vi "γ能量测量实验.vi"() -> ()   [LabVIEW 2014]
panel:
  in  "放大倍数":dbl min=0.0 max=2.0
  in  "按钮_提示":bool caption="提示"
  in  "选项卡控件 实验步骤":T1(tab)
  in  "选项卡控件":enum32{"选项卡 3", "选项卡 1", "选项卡 2", "选项卡 4"}(tab)
  in  "放射源":string(combo)
  in  "按钮_退出":bool
  in  "按钮_开始测量":bool
  in  "按钮_加载高压":bool
  in  "按钮_放置放射源":bool
  in  "按钮_打开多道":bool
  out "高压输入":bool
  out "0-1KV":dbl(knob) scale=0.0..1.0
  out "信号输出指示":bool caption="信号输出"
  in  "按钮_恢复仪器状态":bool
  out "退出":bool
  out "信号输出":bool
  out "是否放置放射源":bool
  in  "脉冲间隔时间":i16
  in  "数组_各放射源初始计数率":dbl[](array[numeric])
  # "实验：γ能谱测量实验"
  # "实验仪器"
  # "实验原理"
  # "实验步骤"
  # "操作面板"
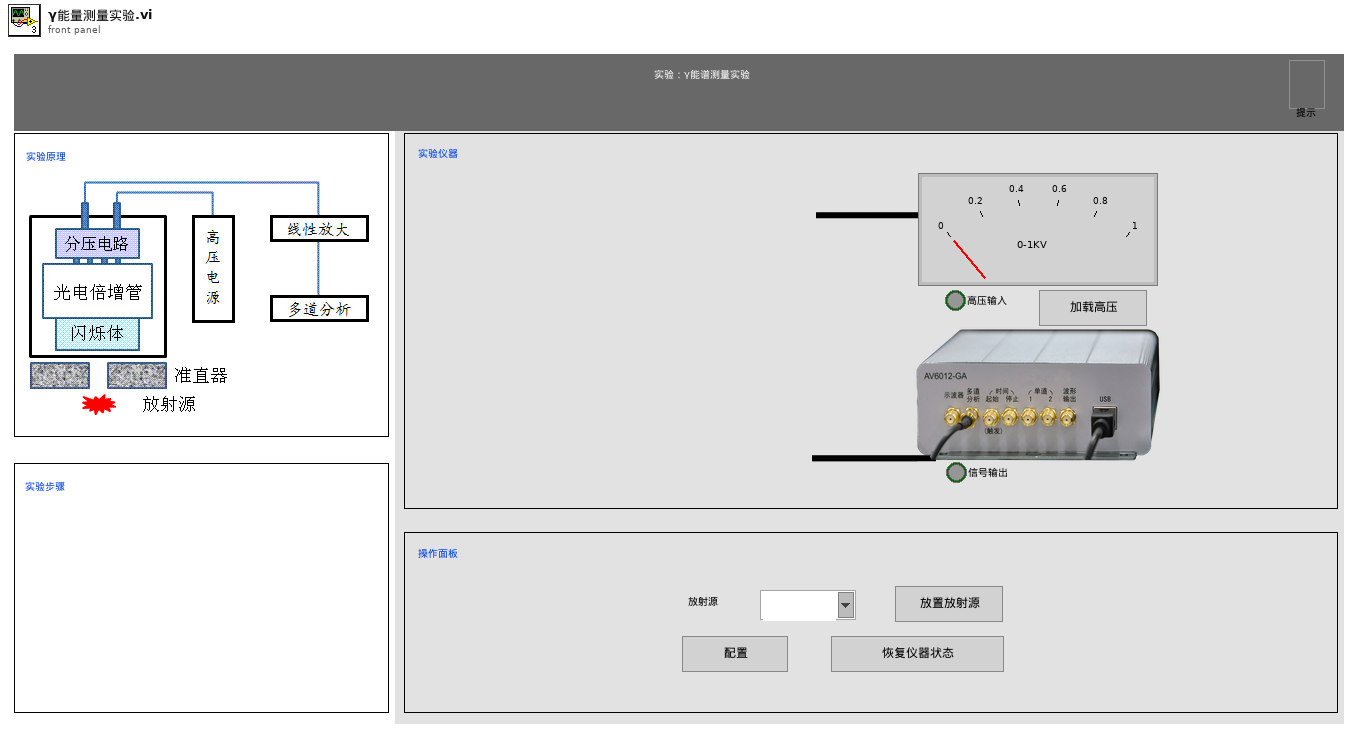
[diagram p1: front panel]
types:
  T1 = enum32{"选项卡 1", "选项卡 2", "选项卡 3", "选项卡 4", "选项卡 5"}
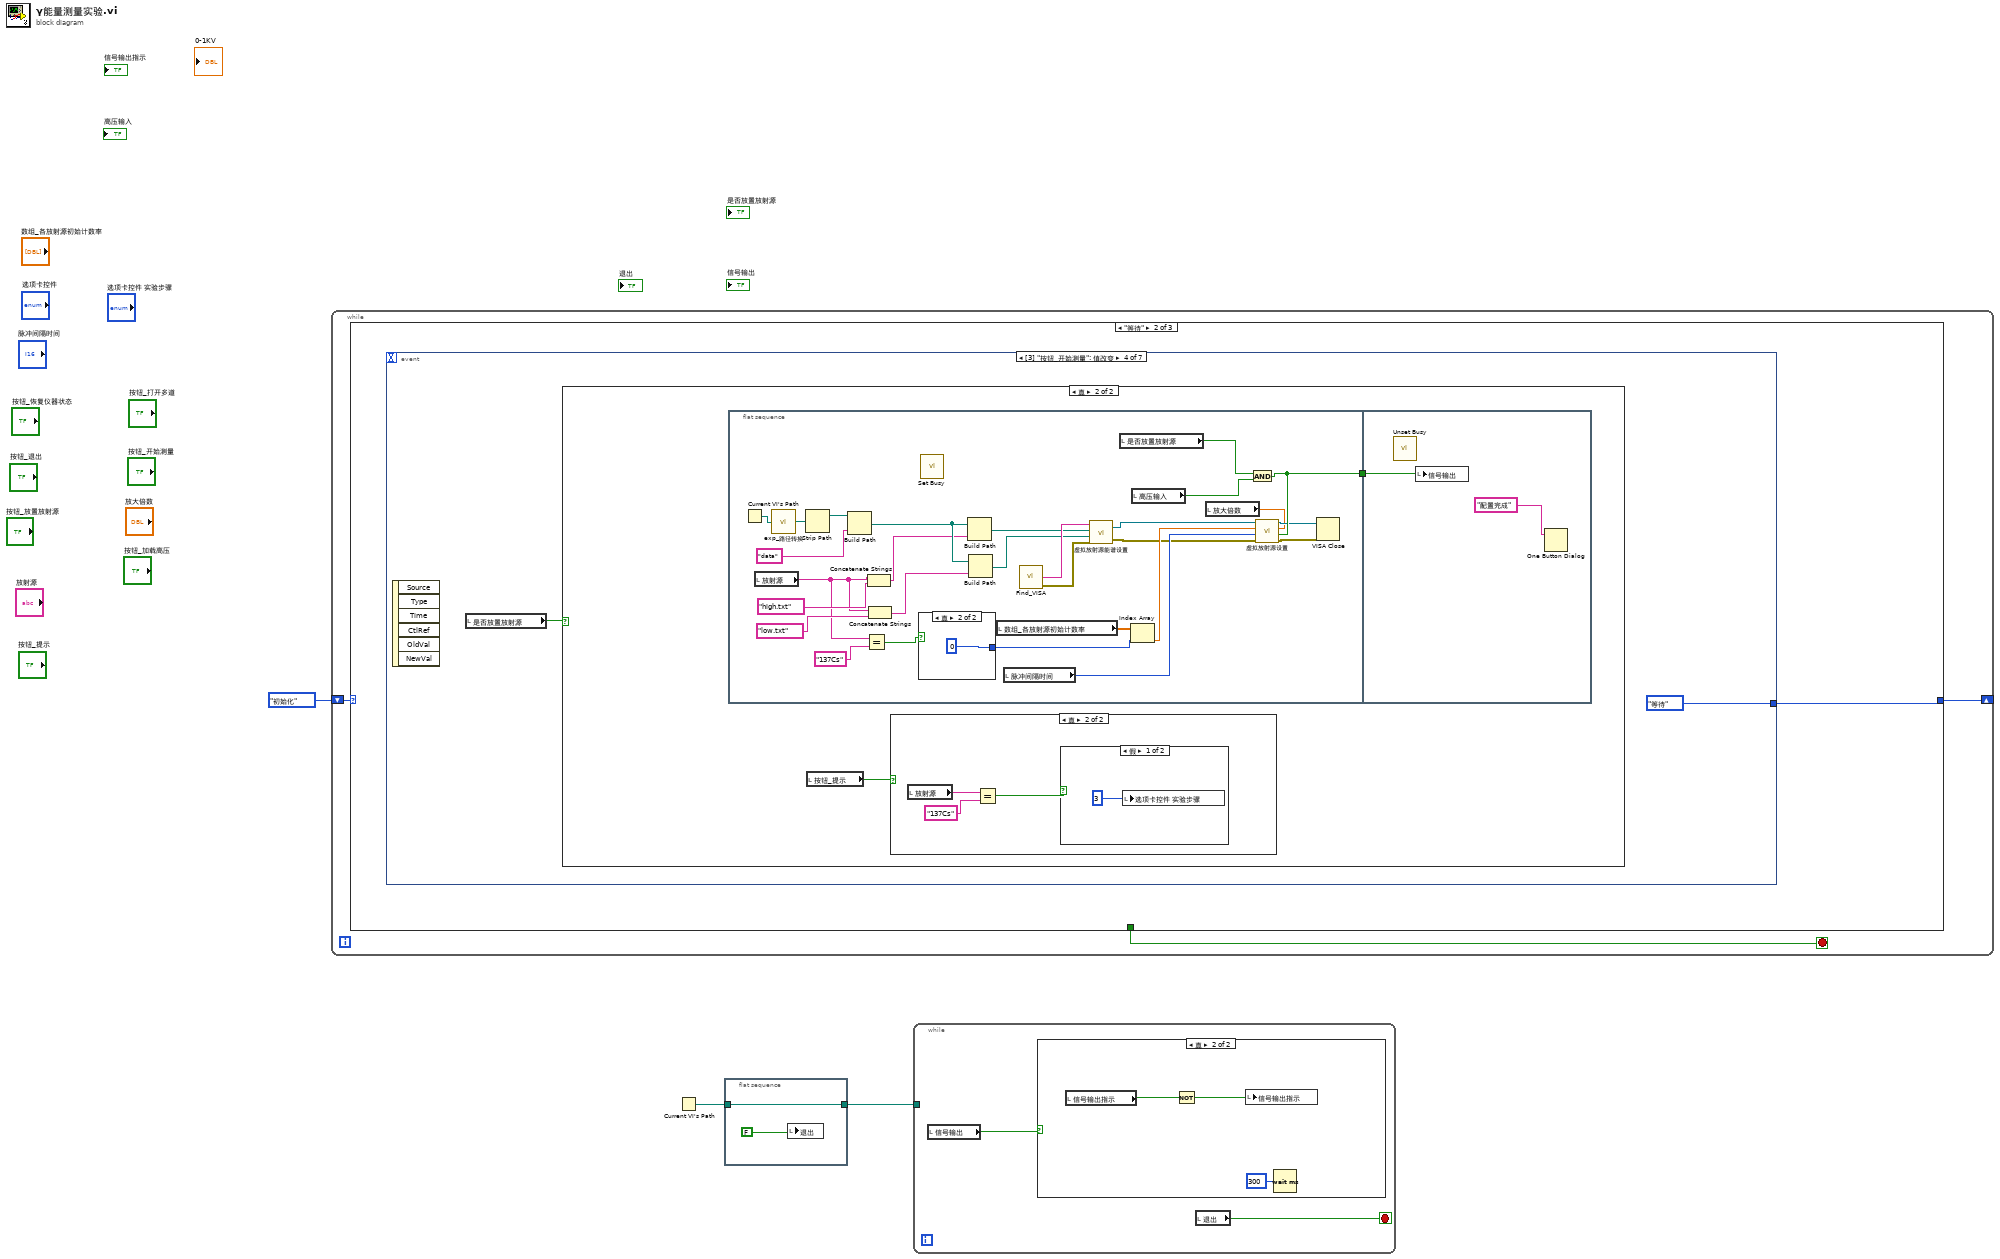
[diagram p0: block diagram]
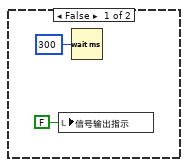
[diagram p2: hidden frame]
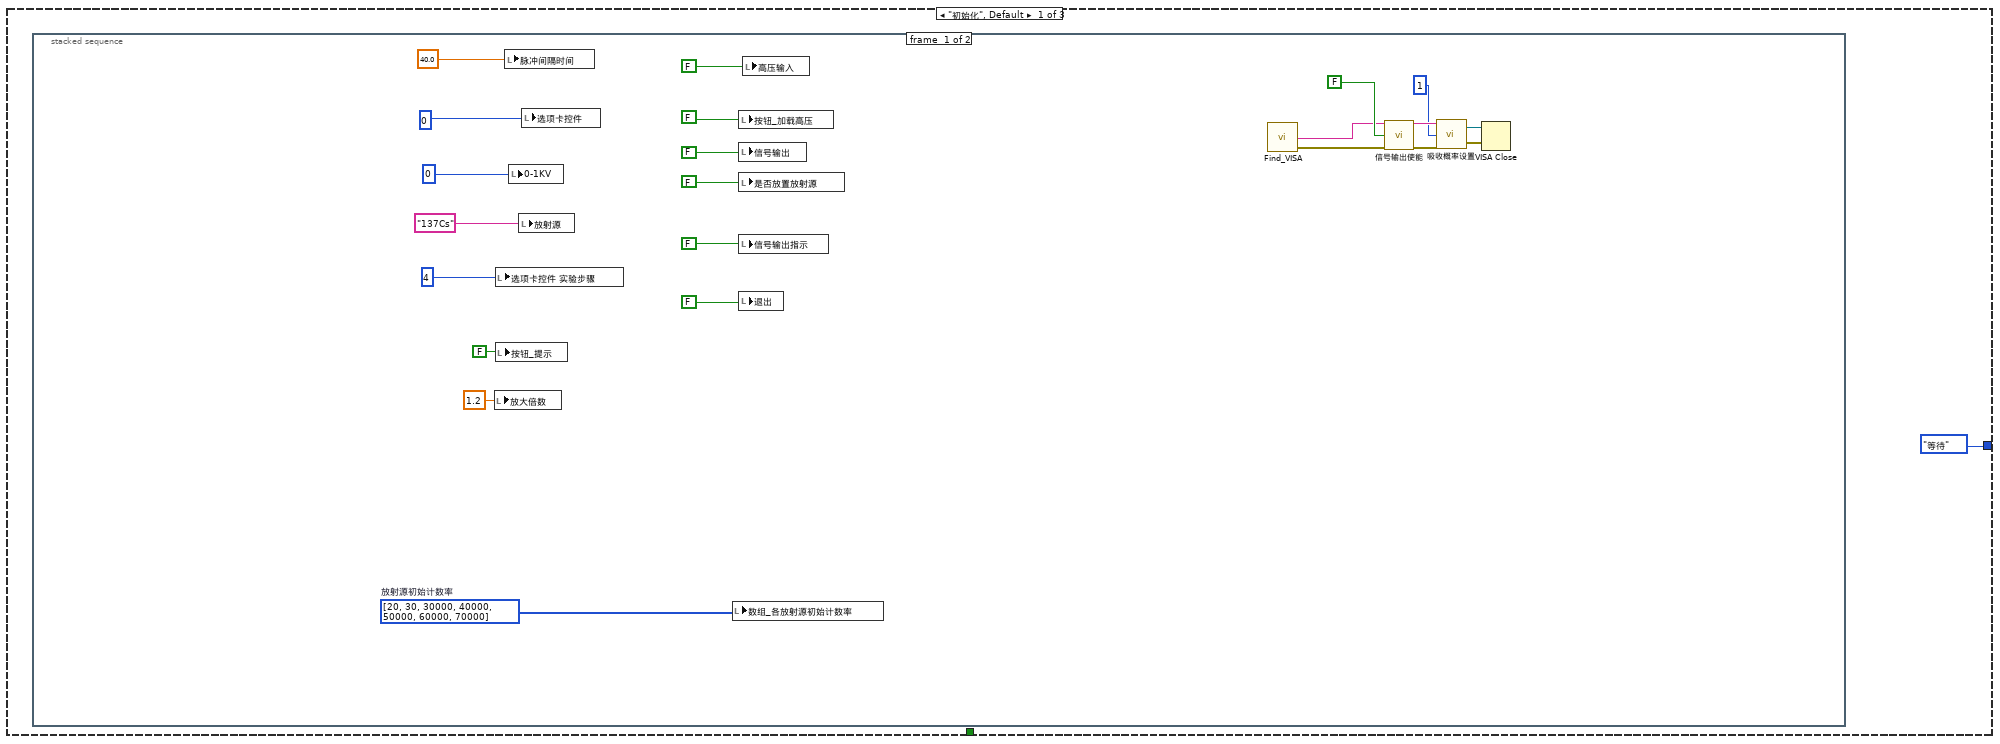
[diagram p3: hidden frame]
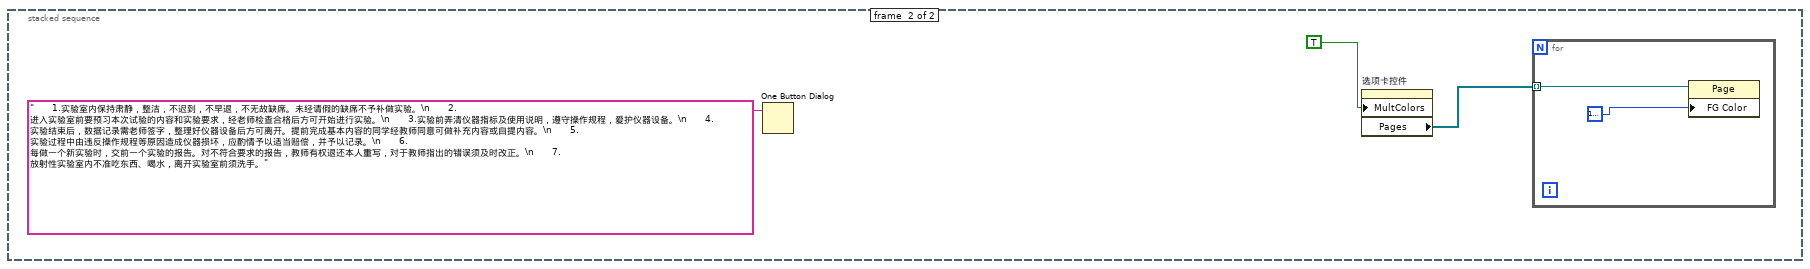
[diagram p4: hidden frame]
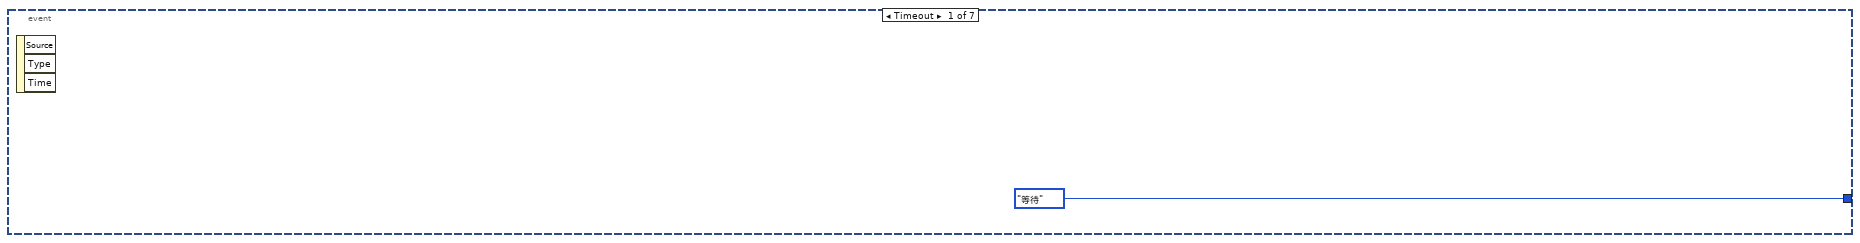
[diagram p5: hidden frame]
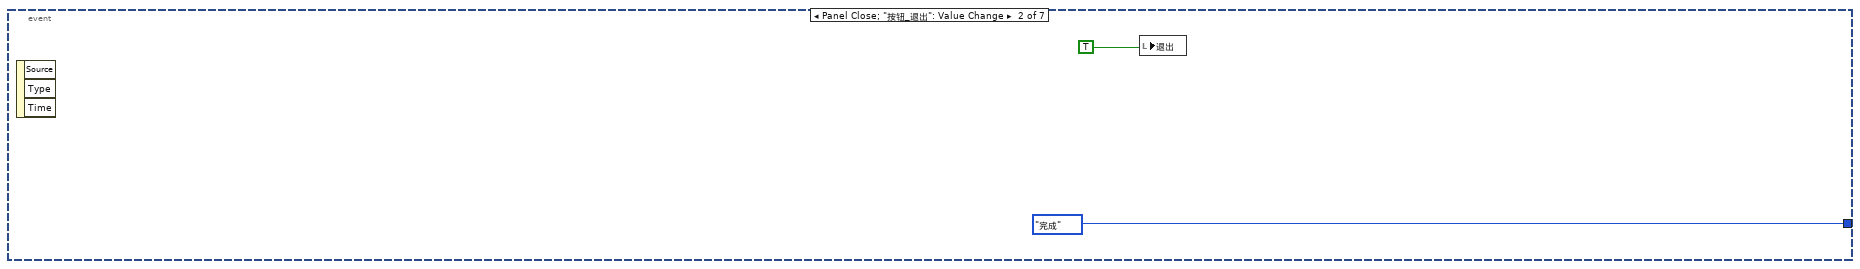
[diagram p6: hidden frame]
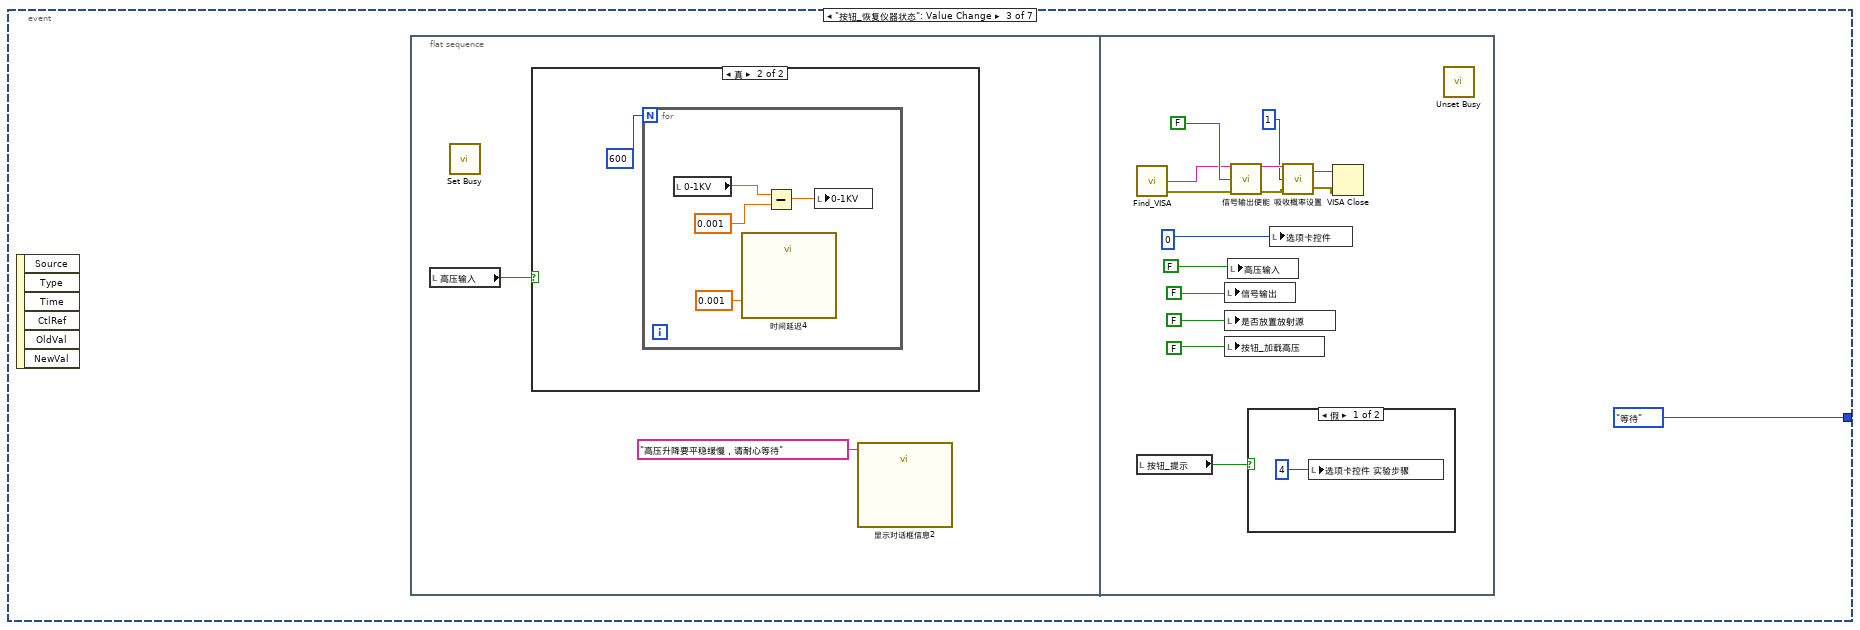
[diagram p7: hidden frame]
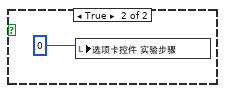
[diagram p9: hidden frame]
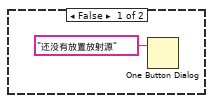
[diagram p10: hidden frame]
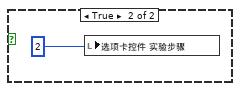
[diagram p12: hidden frame]
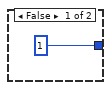
[diagram p13: hidden frame]
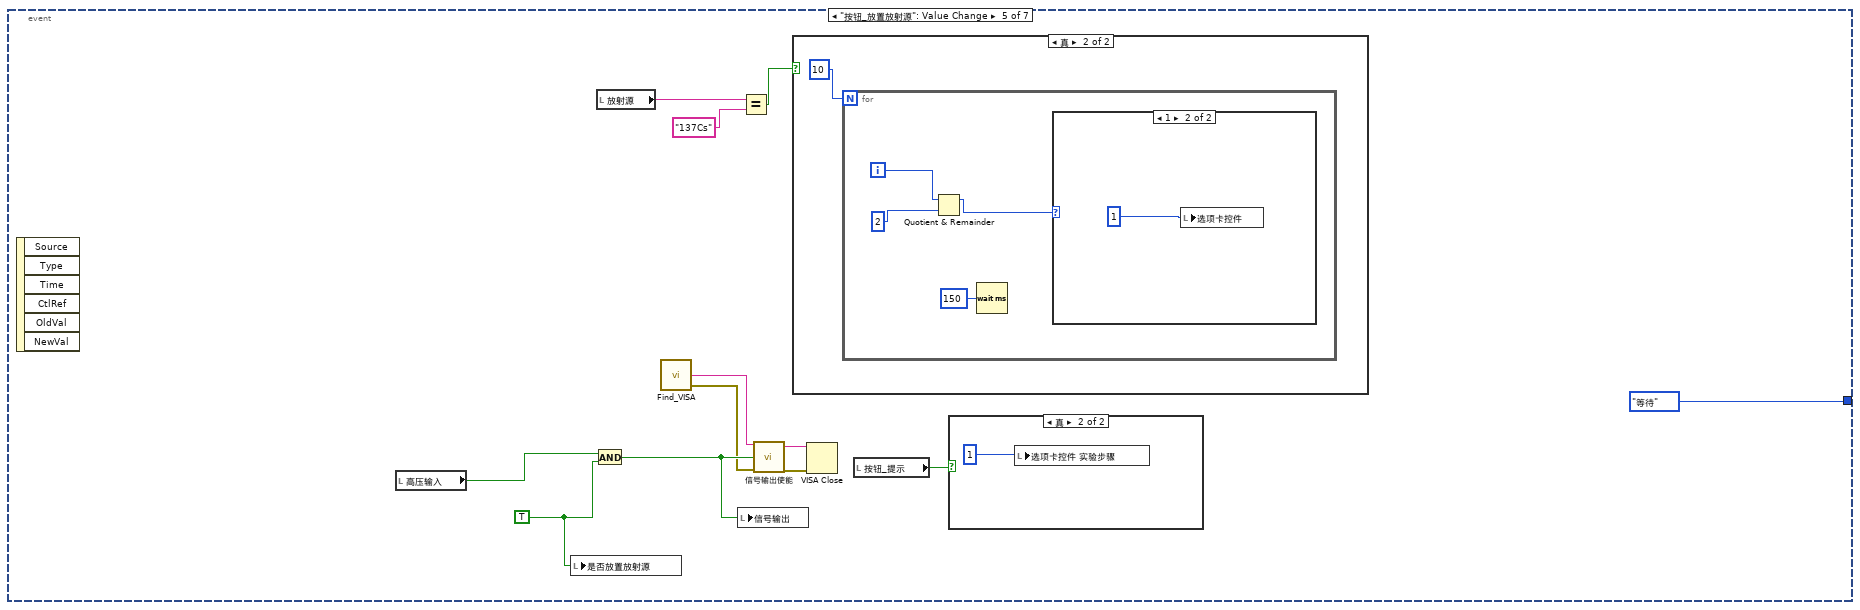
[diagram p14: hidden frame]
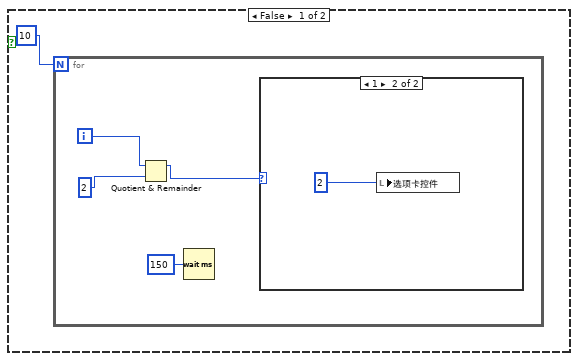
[diagram p16: hidden frame]
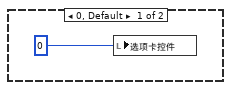
[diagram p17: hidden frame]
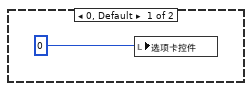
[diagram p18: hidden frame]
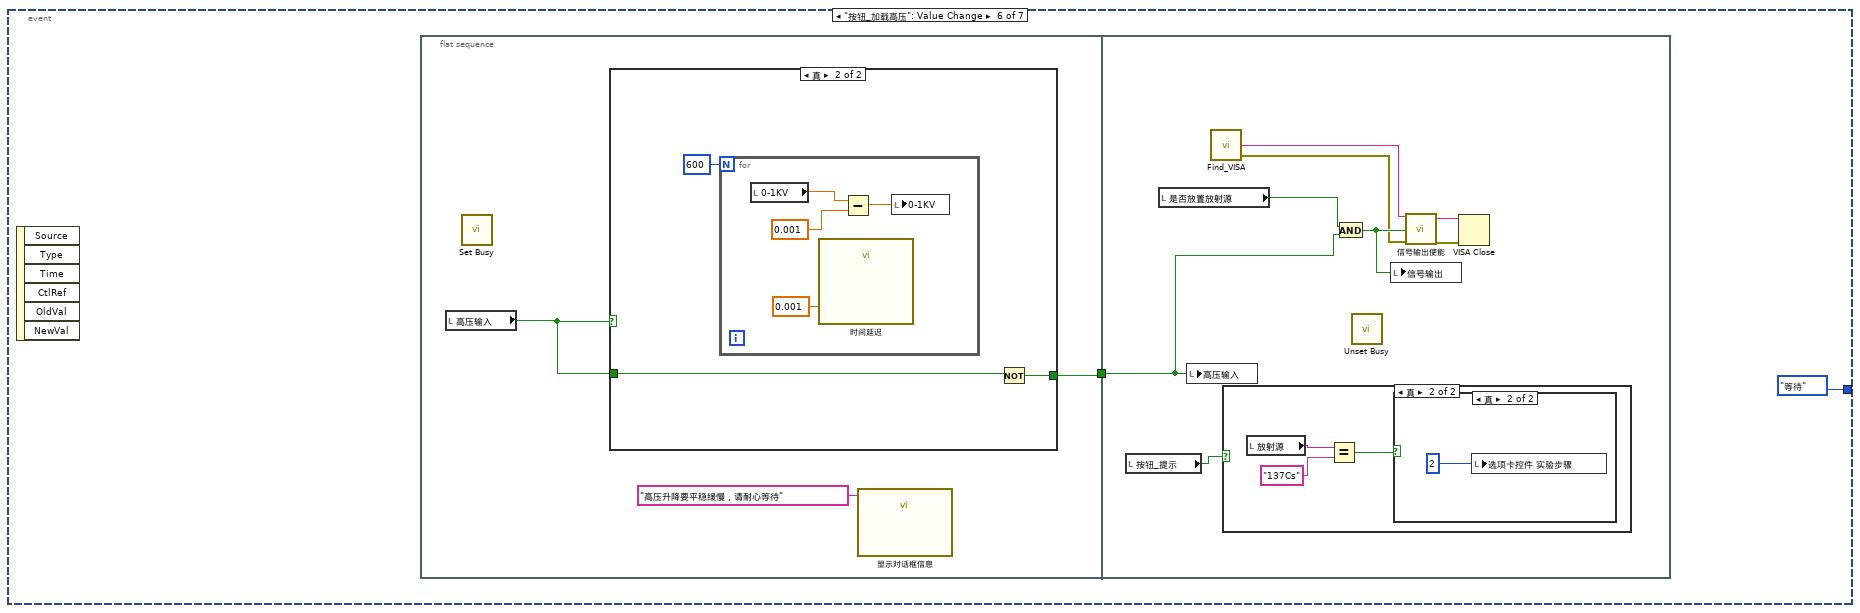
[diagram p19: hidden frame]
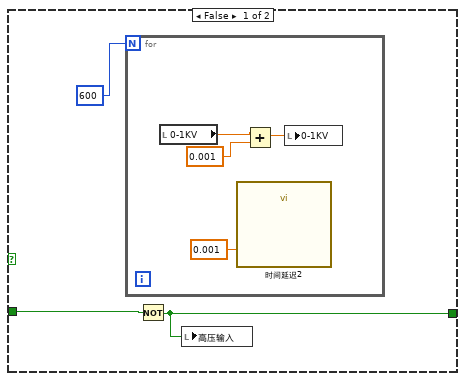
[diagram p20: hidden frame]
diagram:
  n1 = while {
    shift-right: [w5] -> _
    shift-left: enum16{"初始化", "等待", "完成"}."初始化" -> [w6]
    stop <- w4 stop-if-true
    n2 = case shown="\"等待\"" w6 {
      tunnel: [enum16{"初始化", "等待", "完成"}."等待" w35 enum16{"初始化", "等待", "完成"}."完成"] -> w5
      tunnel: [_ _ TRUE] -> w4
      frame "初始化", Default {
        n3 = stacked-sequence {
          frame #0 {
            w28 = i32[] [20, 30, 30000, 40000, 50000, 60000, 70000]  # 放射源初始计数率
            n4 = local write "放大倍数"(1.2 ("放大倍数")) -> ()
            n5 = local write "选项卡控件 实验步骤"(4) -> ()
            n6 = local write "按钮_提示"(FALSE ("按钮_提示")) -> ()
            n7 = local write "脉冲间隔时间"(40.0 ("脉冲间隔时间")) -> ()
            n8 = local write "0-1KV"(0) -> ()
            n9 = local write "放射源"("137Cs") -> ()
            n10 = local write "选项卡控件"(0) -> ()
            n11 = local write "数组_各放射源初始计数率"(w28) -> ()
            n12 = local write "按钮_加载高压"(FALSE ("高压开关")) -> ()
            n13 = local write "信号输出"(FALSE ("高压开关")) -> ()
            n14 = local write "是否放置放射源"(FALSE ("高压开关")) -> ()
            n15 = local write "信号输出指示"(FALSE ("高压开关")) -> ()
            n16 = local write "退出"(FALSE ("高压开关")) -> ()
            n17 = local write "高压输入"(FALSE ("高压开关")) -> ()
            n18 = call "Find_VISA.vi"() -> ("错误输出"=w17:errorcluster, "虚拟放射源VISA"=w18:string)  [unwired: 3 in, 1 out]
            n19 = call "信号输出使能.vi"("VISA资源名称"=w18, "信号输出"=FALSE, "错误输入（无错误）"=w17) -> ("元素 2"=w16:string, "错误输出 2"=w14:errorcluster)  [unwired: 11 in]
            n20 = call "吸收概率设置.vi"("错误输入（无错误）"=w14, "衰减"=u16 1 ("衰减倍数"), "VISA资源名称"=w16) -> ("错误输出"=w12:errorcluster, "VISA资源名称输出"=w13:refnum<visa-resource-name>)
            n21 = VISA Close(VISA resource name=w13, error in (no error)=w12) -> ()  [unwired: 1 out]
          }
          frame #1 {
            n22 = One Button Dialog(message="      1.实验室内保持肃静，整洁，不迟到，不早退，不无故缺席。未经请假的缺席不予补做实验。\n      2.进入实验室前要预习本次试验的内容和实验要求，经老师检查合格后方可开始进行实验。\n      3.实验前弄清仪器指标及使用说明，遵守操作规程，爱护仪器设备。\n      4.实验结束后，数据记录需老师签字，整理好仪器设备后方可离开。提前完成基本内容的同学经教师同意可做补充内容或自提内容。\n      5.实验过程中由违反操作规程等原因造成仪器损坏，应酌情予以适当赔偿，并予以记录。\n      6.每做一个新实验时，交前一个实验的报告。对不符合要求的报告，教师有权退还本人重写，对于教师指出的错误须及时改正。\n      7.放射性实验室内不准吃东西、喝水，离开实验室前须洗手。" ("消息")) -> ()  [unwired: 1 in, 1 out]
            n23 = property on="选项卡控件" class="TabCtl (严格)"("MultColors"=TRUE ("允许多种颜色")) -> ("Pages"=w31:refnum<vi>[])  [unwired: 2 in, 2 out]
            n24 = for {
              tunnel: w31 -> [w34] mode=indexing
              n25 = property class="Page"(reference=w34, "FG Color"=u32 16777216) -> ()  [unwired: 1 in, 2 out]
            }
          }
        }
      }
      frame "等待" {
        n26 = event shown="[3] \"按钮_开始测量\": 值改变" {
          selector: _ -> [_ _ _ _ _ _ _]
          dyn-events: _ -> [_ _ _ _ _ _ _]
          timeout: _ -> [_ _ _ _ _ _ _]
          tunnel: [enum16{"初始化", "等待", "完成"}."等待" enum16{"初始化", "等待", "完成"}."完成" enum16{"初始化", "等待", "完成"}."等待" enum16{"初始化", "等待", "完成"}."等待" enum16{"初始化", "等待", "完成"}."等待" enum16{"初始化", "等待", "完成"}."等待" enum16{"初始化", "等待", "完成"}."等待"] -> w35
          event Timeout {
            n27 = event-data() -> ()  [unwired: 1 in, 3 out]
          }
          event Panel Close; "按钮_退出": Value Change {
            n28 = event-data() -> ()  [unwired: 1 in, 3 out]
            n29 = local write "退出"(TRUE ("高压开关")) -> ()
          }
          event "按钮_恢复仪器状态": Value Change {
            n30 = event-data() -> ()  [unwired: 1 in, 6 out]
            n31 = flat-sequence {
              frame #0 {
                n32 = local read "高压输入"() -> (w40:bool)
                n33 = call <vilib>:"Set Busy.vi"() -> ()  [unwired: 10 in, 2 out]
                n34 = case shown="真" w40 {
                  frame False {
                  }
                  frame True {
                    n35 = for {
                      N: 600 -> [_]
                      n36 = local read "0-1KV"() -> (w45:dbl)
                      n37 = call "时间延迟4"("Delay Time (s)"=0.001) -> ()  [unwired: 10 in, 1 out]
                      n38 = Subtract(x=w45, y=0.001) -> (x-y=w43:dbl)
                      n39 = local write "0-1KV"(w43) -> ()
                    }
                  }
                }
                n40 = call "显示对话框信息2"("Message"="高压升降要平稳缓慢，请耐心等待") -> ()  [unwired: 9 in, 2 out]
              }
              frame #1 {
                n41 = call "Find_VISA.vi"() -> ("错误输出"=w54:errorcluster, "虚拟放射源VISA"=w55:string)  [unwired: 3 in, 1 out]
                n42 = local read "按钮_提示"() -> (w47:bool)
                n43 = local write "信号输出"(FALSE ("高压开关")) -> ()
                n44 = local write "是否放置放射源"(FALSE ("高压开关")) -> ()
                n45 = local write "按钮_加载高压"(FALSE ("高压开关")) -> ()
                n46 = local write "高压输入"(FALSE ("高压开关")) -> ()
                n47 = call "信号输出使能.vi"("VISA资源名称"=w55, "信号输出"=FALSE, "错误输入（无错误）"=w54) -> ("元素 2"=w53:string, "错误输出 2"=w52:errorcluster)  [unwired: 11 in]
                n48 = case shown="假" w47 {
                  frame False {
                    n49 = local write "选项卡控件 实验步骤"(4) -> ()
                  }
                  frame True {
                    n50 = local write "选项卡控件 实验步骤"(0) -> ()
                  }
                }
                n51 = local write "选项卡控件"(0) -> ()
                n52 = call "吸收概率设置.vi"("错误输入（无错误）"=w52, "衰减"=u16 1, "VISA资源名称"=w53) -> ("错误输出"=w50:errorcluster, "VISA资源名称输出"=w51:refnum<visa-resource-name>)
                n53 = VISA Close(VISA resource name=w51, error in (no error)=w50) -> ()  [unwired: 1 out]
                n54 = call <vilib>:"Unset Busy.vi"() -> ()  [unwired: 11 in, 1 out]
              }
            }
          }
          event "按钮_开始测量": Value Change {
            n55 = event-data() -> ()  [unwired: 1 in, 6 out]
            n56 = local read "是否放置放射源"() -> (w63:bool)
            n57 = case shown="真" w63 {
              frame False {
                n58 = One Button Dialog(message="还没有放置放射源" ("消息")) -> ()  [unwired: 1 in, 1 out]
              }
              frame True {
                n59 = flat-sequence {
                  tunnel: [w77] -> w67
                  tunnel: w67 -> [w104]
                  frame #0 {
                    n60 = Current VI's Path() -> (path=w73:path)
                    n61 = local read "放射源"() -> (w87:string)
                    n62 = call "exp_路径转换.vi"("input path"=w73) -> ("output path"=w74:path)
                    n63 = Strip Path(path=w74) -> (stripped path=w99:path)  [unwired: 1 out]
                    n64 = Build Path(base path=w99, name or relative path="data") -> (appended path=w98:path)
                    n65 = Equal?(x=w87, y="137Cs") -> (x = y?=w85:bool)
                    n66 = Concatenate Strings(w87, "high.txt") -> (w89:string)
                    n67 = Concatenate Strings(w87, "low.txt") -> (w88:string)
                    n68 = case shown="真" w85 {
                      tunnel: [1 0] -> w84
                      frame False {
                      }
                      frame True {
                      }
                    }
                    n69 = call <vilib>:"Set Busy.vi"() -> ()  [unwired: 10 in, 2 out]
                    n70 = Build Path(base path=w98, name or relative path=w89) -> (appended path=w94:path)
                    n71 = Build Path(base path=w98, name or relative path=w88) -> (appended path=w93:path)
                    n72 = local read "数组_各放射源初始计数率"() -> (w97:dbl[])
                    n73 = local read "脉冲间隔时间"() -> (w80:i16)
                    n74 = call "Find_VISA.vi"() -> ("错误输出"=w92:errorcluster, "虚拟放射源VISA"=w95:string)  [unwired: 3 in, 1 out]
                    n75 = call "虚拟放射源能谱设置.vi"("错误输入（无错误）"=w92, "低位数据路径"=w93, "高位数据路径"=w94, "VISA资源名称"=w95) -> ("错误输出"=w79:errorcluster, "VISA资源名称输出"=w82:refnum<visa-resource-name>)
                    n76 = local read "是否放置放射源"() -> (w83:bool)
                    n77 = Index Array(array=w97, index=w84) -> (element=w81:dbl)
                    n78 = local read "高压输入"() -> (w96:bool)
                    n79 = local read "放大倍数"() -> (w75:dbl)
                    n80 = And(x=w83, y=w96) -> (x .and. y?=w77:bool)
                    n81 = call "虚拟放射源设置.vi"("信号输出"=w77, "放大倍数"=w75, "错误输入（无错误）"=w79, "最小时间间隔"=w80, "计数率"=w81, "VISA资源名称"=w82) -> ("错误输出"=w78:errorcluster, "VISA资源名称输出"=w76:refnum<visa-resource-name>)
                    n82 = VISA Close(VISA resource name=w76, error in (no error)=w78) -> ()  [unwired: 1 out]
                  }
                  frame #1 {
                    n83 = call <vilib>:"Unset Busy.vi"() -> ()  [unwired: 11 in, 1 out]
                    n84 = local write "信号输出"(w104) -> ()
                    n85 = One Button Dialog(message="配置完成") -> ()  [unwired: 1 in, 1 out]
                  }
                }
                n86 = local read "按钮_提示"() -> (w66:bool)
                n87 = case shown="真" w66 {
                  frame False {
                  }
                  frame True {
                    n88 = local read "放射源"() -> (w69:string)
                    n89 = Equal?(x=w69, y="137Cs") -> (x = y?=w68:bool)
                    n90 = case shown="假" w68 {
                      frame False {
                        n91 = local write "选项卡控件 实验步骤"(3) -> ()
                      }
                      frame True {
                        n92 = local write "选项卡控件 实验步骤"(2) -> ()
                      }
                    }
                  }
                }
              }
            }
          }
          event "按钮_放置放射源": Value Change {
            w113 = TRUE
            n93 = event-data() -> ()  [unwired: 1 in, 6 out]
            n94 = local read "高压输入"() -> (w106:bool)
            n95 = local write "是否放置放射源"(w113) -> ()
            n96 = And(x=w106, y=w113) -> (x .and. y?=w112:bool)
            n97 = local read "放射源"() -> (w108:string)
            n98 = call "Find_VISA.vi"() -> ("错误输出"=w110:errorcluster, "虚拟放射源VISA"=w111:string)  [unwired: 3 in, 1 out]
            n99 = local write "信号输出"(w112) -> ()
            n100 = Equal?(x=w108, y="137Cs") -> (x = y?=w107:bool)
            n101 = call "信号输出使能.vi"("VISA资源名称"=w111, "信号输出"=w112, "错误输入（无错误）"=w110) -> ("元素 2"=w115:string, "错误输出 2"=w114:errorcluster)  [unwired: 11 in]
            n102 = case shown="真" w107 {
              frame False {
                n103 = for {
                  N: 10 -> [_]
                  i -> [w122]
                  n104 = Quotient & Remainder(x=w122, y=2) -> (x-y*floor(x/y)=w120:i32)  [unwired: 1 out]
                  n105 = Wait (ms)(milliseconds to wait=u32 150 ("等待时间（毫秒）")) -> ()  [unwired: 1 out]
                  n106 = case shown="1" w120 {
                    frame 0, Default {
                      n107 = local write "选项卡控件"(0) -> ()
                    }
                    frame 1 {
                      n108 = local write "选项卡控件"(2) -> ()
                    }
                  }
                }
              }
              frame True {
                n109 = for {
                  N: 10 -> [_]
                  i -> [w129]
                  n110 = Quotient & Remainder(x=w129, y=2) -> (x-y*floor(x/y)=w127:i32)  [unwired: 1 out]
                  n111 = Wait (ms)(milliseconds to wait=u32 150 ("等待时间（毫秒）")) -> ()  [unwired: 1 out]
                  n112 = case shown="1" w127 {
                    frame 0, Default {
                      n113 = local write "选项卡控件"(0) -> ()
                    }
                    frame 1 {
                      n114 = local write "选项卡控件"(1) -> ()
                    }
                  }
                }
              }
            }
            n115 = VISA Close(VISA resource name=w115, error in (no error)=w114) -> ()  [unwired: 1 out]
            n116 = local read "按钮_提示"() -> (w105:bool)
            n117 = case shown="真" w105 {
              frame False {
              }
              frame True {
                n118 = local write "选项卡控件 实验步骤"(1) -> ()
              }
            }
          }
          event "按钮_加载高压": Value Change {
            n119 = event-data() -> ()  [unwired: 1 in, 6 out]
            n120 = flat-sequence {
              tunnel: [w134] -> w132
              tunnel: w132 -> [w155]
              frame #0 {
                n121 = local read "高压输入"() -> (w136:bool)
                n122 = call <vilib>:"Set Busy.vi"() -> ()  [unwired: 10 in, 2 out]
                n123 = case shown="真" w136 {
                  tunnel: w136 -> [w138 w145]
                  tunnel: [w137 w144] -> w134
                  frame False {
                    n124 = for {
                      N: 600 -> [_]
                      n125 = local read "0-1KV"() -> (w142:dbl)
                      n126 = call "时间延迟2"("Delay Time (s)"=0.001) -> ()  [unwired: 10 in, 1 out]
                      n127 = Add(x=w142, y=0.001) -> (x+y=w143:dbl)
                      n128 = local write "0-1KV"(w143) -> ()
                    }
                    n129 = Not(x=w138) -> (.not. x?=w137:bool)
                    n130 = local write "高压输入"(w137) -> ()
                  }
                  frame True {
                    n131 = for {
                      N: 600 -> [_]
                      n132 = local read "0-1KV"() -> (w149:dbl)
                      n133 = call "时间延迟"("Delay Time (s)"=0.001) -> ()  [unwired: 10 in, 1 out]
                      n134 = Subtract(x=w149, y=0.001) -> (x-y=w147:dbl)
                      n135 = local write "0-1KV"(w147) -> ()
                    }
                    n136 = Not(x=w145) -> (.not. x?=w144:bool)
                  }
                }
                n137 = call "显示对话框信息"("Message"="高压升降要平稳缓慢，请耐心等待") -> ()  [unwired: 9 in, 2 out]
              }
              frame #1 {
                n138 = local read "按钮_提示"() -> (w151:bool)
                n139 = local read "是否放置放射源"() -> (w152:bool)
                n140 = local write "高压输入"(w155) -> ()
                n141 = call "Find_VISA.vi"() -> ("错误输出"=w153:errorcluster, "虚拟放射源VISA"=w154:string)  [unwired: 3 in, 1 out]
                n142 = case shown="真" w151 {
                  frame False {
                  }
                  frame True {
                    n143 = local read "放射源"() -> (w160:string)
                    n144 = Equal?(x=w160, y="137Cs") -> (x = y?=w159:bool)
                    n145 = case shown="真" w159 {
                      frame False {
                        n146 = local write "选项卡控件 实验步骤"(3) -> ()
                      }
                      frame True {
                        n147 = local write "选项卡控件 实验步骤"(2) -> ()
                      }
                    }
                  }
                }
                n148 = And(x=w152, y=w155) -> (x .and. y?=w156:bool)
                n149 = call <vilib>:"Unset Busy.vi"() -> ()  [unwired: 11 in, 1 out]
                n150 = local write "信号输出"(w156) -> ()
                n151 = call "信号输出使能.vi"("VISA资源名称"=w154, "信号输出"=w156, "错误输入（无错误）"=w153) -> ("元素 2"=w158:string, "错误输出 2"=w157:errorcluster)  [unwired: 11 in]
                n152 = VISA Close(VISA resource name=w158, error in (no error)=w157) -> ()  [unwired: 1 out]
              }
            }
          }
          event "按钮_提示": Value Change {
            n153 = event-data() -> ()  [unwired: 1 in, 6 out]
            n154 = local read "按钮_提示"() -> (w165:bool)
            n155 = case shown="真" w165 {
              frame False {
                n156 = local write "选项卡控件 实验步骤"(T1."选项卡 5" ("选项卡控件 实验步骤")) -> ()
              }
              frame True {
                n157 = local read "是否放置放射源"() -> (w167:bool)
                n158 = case shown="真" w167 {
                  frame False {
                    n159 = local write "选项卡控件 实验步骤"(T1."选项卡 1" ("选项卡控件 实验步骤")) -> ()
                  }
                  frame True {
                    n160 = local read "按钮_加载高压"() -> (w169:bool)
                    n161 = case shown="真" w169 {
                      frame False {
                        n162 = local write "选项卡控件 实验步骤"(T1."选项卡 2" ("选项卡控件 实验步骤")) -> ()
                      }
                      frame True {
                        n163 = local read "放射源"() -> (w172:string)
                        n164 = Equal?(x=w172, y="137Cs") -> (x = y?=w171:bool)
                        n165 = case shown="真" w171 {
                          frame False {
                            n166 = local write "选项卡控件 实验步骤"(T1."选项卡 4" ("选项卡控件 实验步骤")) -> ()
                          }
                          frame True {
                            n167 = local write "选项卡控件 实验步骤"(T1."选项卡 3" ("选项卡控件 实验步骤")) -> ()
                          }
                        }
                      }
                    }
                  }
                }
              }
            }
          }
        }
      }
      frame "完成" {
      }
    }
  }
  n168 = Current VI's Path() -> (path=w2:path)
  n169 = flat-sequence {
    tunnel: w2 -> [w178]
    tunnel: [w178] -> w1
    frame #0 {
      n170 = local write "退出"(FALSE ("高压开关")) -> ()
    }
  }
  n171 = while {
    tunnel: w1 -> [_]
    stop <- w180 stop-if-true
    n172 = local read "信号输出"() -> (w181:bool)
    n173 = case shown="真" w181 {
      frame False {
        n174 = local write "信号输出指示"(FALSE ("信号输出指示")) -> ()
        n175 = Wait (ms)(milliseconds to wait=u32 300 ("等待时间（毫秒）")) -> ()  [unwired: 1 out]
      }
      frame True {
        n176 = local read "信号输出指示"() -> (w186:bool)
        n177 = Not(x=w186) -> (.not. x?=w185:bool)
        n178 = local write "信号输出指示"(w185) -> ()
        n179 = Wait (ms)(milliseconds to wait=u32 300 ("等待时间（毫秒）")) -> ()  [unwired: 1 out]
      }
    }
    n180 = local read "退出"() -> (w180:bool)
  }
